vi "Player Info.vi"(11 "Concentricity in":refnum<class "Base Builder.lvclass">) -> (1 "Victory Speech":string, 2 "Name":string, 3 "Concentricity out":refnum<class "Base Builder.lvclass">)   [LabVIEW 2015, in "Base Builder.lvclass"]
uses:
  Base Builder/Base Builder.lvclass
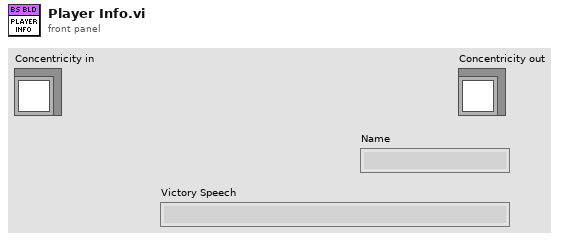
[diagram p1: front panel]
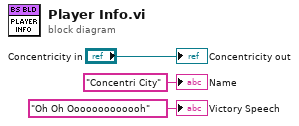
[diagram p0: block diagram]
diagram:
  "Concentricity out" <- "Concentricity in"
  "Name" <- "Concentri City" ("Name")
  "Victory Speech" <- "Oh Oh Ooooooooooooh" ("Victory Speech")
